vi "Open Log Reference.vi"(11 "Project Path":path) -> (0 "error out":errorcluster, 3 "File Reference":refnum<file>)   [LabVIEW 2016, in "PantherLAB_Scripting.lvlib"]
uses:
  PantherLAB_Scripting.lvlib
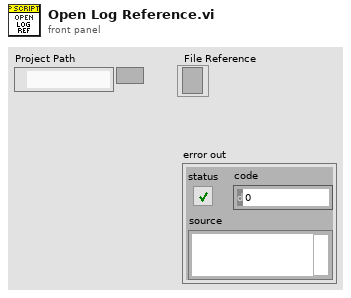
[diagram p1: front panel]
types:
  T1 = enum16{"open", "replace", "create", "open or create", "replace or create", "replace or create with confirmation"}
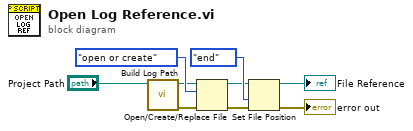
[diagram p0: block diagram]
diagram:
  n1 = call "Build Log Path.vi"("Project Path"="Project Path") -> ("error out"=w9:errorcluster, "PantherLAB Log File Path"=w1:path)  [unwired: 9 in]
  n2 = Open/Create/Replace File(file path (use dialog)=w1, error in=w9, operation (0:open)=T1."open or create") -> (refnum out=w3:refnum<file>, error out=w7:errorcluster)  [unwired: 3 in, 1 out]
  n3 = Set File Position(refnum=w3, from (0:start)=enum16{"start", "end", "current"}."end", error in=w7) -> (refnum out=→"File Reference":refnum<file>, error out=→"error out":errorcluster)  [unwired: 1 in]
